vi "climber_calc.vi"(11 "Climber_Commands":T2) -> (3 "Climber_Outputs":T1)   [LabVIEW 2012]
uses:
  climber_cmds.ctl
  climber_outputs.ctl
panel:
  in  "Climber_Outputs 2":T1
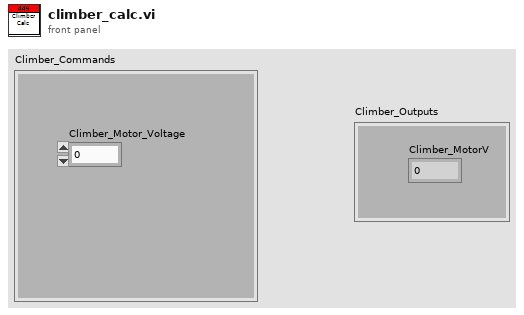
[diagram p1: front panel]
types:
  T1 = typedef "climber_outputs.ctl" = cluster{"Climber_MotorV":dbl}
  T2 = typedef "climber_cmds.ctl" = cluster{"Climber_Motor_Voltage":dbl}
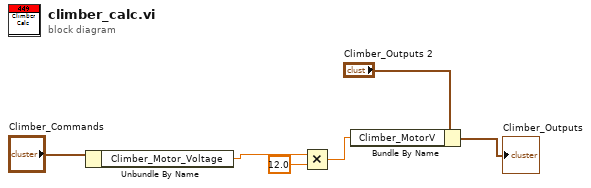
[diagram p0: block diagram]
diagram:
  n1 = Unbundle By Name("Climber_Commands") -> ("Climber_Motor_Voltage"=w5:dbl)
  n2 = Multiply(x=w5, y=12.0) -> (x*y=w2:dbl)
  n3 = Bundle By Name(cluster="Climber_Outputs 2", "Climber_MotorV"=w2) -> (→"Climber_Outputs":T1)
